vi "2D_voltage_mapping_lock-in-measurement_11_25_24.vi"() -> ()   [LabVIEW 2024]
uses:
  <vilib>/Utility/file.llb/Write Delimited Spreadsheet (string).vi
  <vilib>/Utility/file.llb/Write Delimited Spreadsheet (DBL).vi
  C:/Users/Public/OneDrive/Desktop/Keithley_2450_2470_1_4_0_LV2015_NewReadme2_2450-LV2015-1.4.0/Keithley 2450/Keithley 2450.lvlib
  archive/Keithley 24XX/Keithley 24XX.lvlib
  <vilib>/Analysis/NI_AALBase.lvlib
panel:
  out "current set voltage 2410":dbl
  out "Current set voltage 2450":dbl
  out "current voltage 2410":dbl=-5.417298089014366e-05 format="%0.4f"
  out "standard deviation current measured 2410":dbl=4.144039636185763e-09 format="%0.5e"
  out "mean current measured 2410":dbl=-4.484183666747521e-10 format="%0.5e"
  out "current voltage 2450":dbl=-2.554264496e-05 format="%0.4f"
  out "mean current measured 2450":dbl=-1.909496952e-09 format="%0.5e"
  out "standard deviation current measured 2450":dbl=9.060540822205692e-09 format="%0.5e"
  in  "VISA resource name 2410":refnum<visa-resource-name>="GPIB0::16::INSTR"
  in  "Serial Configuration":T1={"Baud Rate"=9600, "Parity"=0, "Data Bits"=8, "Stop Bits"=10, "Flow Control"=0} {"Flow Control" items=["None", "XON/XOFF", "RTS/CTS", "XON/XOFF & RTS/CTS", "DTR/DSR", "XON/XOFF & DTR/DSR"]; "Stop Bits" items=["1.0"=10, "1.5"=15, "2.0"=20]; "Data Bits" items=["7"=7, "8"=8]; "Parity" items=["None", "Odd", "Even", "Mark", "Space"]; "Baud Rate" items=["300"=300, "600"=600, "1200"=1200, "2400"=2400, "4800"=4800, "9600"=9600, "19200"=19200]}
  in  "Compliance  Level 2410":dbl=5e-08
  in  "Current Num Meas":i32=20 min=1 max=300000 step=1
  in  "VISA resource name 2450":refnum<visa-resource-name>="GPIB0::1::INSTR"
  in  "Current Compliance Limit (0.1) 2450":dbl=5e-08
  in  "ChB Parameter 1":u16(ring)=8 items=["X", "Y", "R", "Theta", "Frequency", "Noise", "Xh1", "Yh1", "Rh1", "Theta h1", "Xh2", "Yh2", "Rh2", "Theta h2"]
  in  "ChB Parameter 2":u16(ring)=9 items=["X", "Y", "R", "Theta", "Frequency", "Noise", "Xh1", "Yh1", "Rh1", "Theta h1", "Xh2", "Yh2", "Rh2", "Theta h2"]
  in  "ChA Parameter 2":u16(ring)=3 items=["X", "Y", "R", "Theta", "Frequency", "Noise", "Xh1", "Yh1", "Rh1", "Theta h1", "Xh2", "Yh2", "Rh2", "Theta h2"]
  in  "ChA Parameter 1":u16(ring)=2 items=["X", "Y", "R", "Theta", "Frequency", "Noise", "Xh1", "Yh1", "Rh1", "Theta h1", "Xh2", "Yh2", "Rh2", "Theta h2"]
  in  "Lock-In Num Avgs":i32=150
  out "错误输出":errorcluster
  in  "OE1022D 2":refnum<visa-resource-name>="COM4" caption="OE1022D"
  in  "ms to wait after move":u32=1000
  in  "Snake":bool
  in  "File to save to":path=path "D:/LabData/XiaoWang_Group_data_2024on/StackingTransitions/CrI3/round5_pfm_dualgate/11-14-4Lsample/RMCD/0T_after_m2T_map.txt"
  in  "Select Scan Type":u16(ring)=1 items=["line scan", "rectangular scan"]
  in  "scan points":i32
  in  "2410 end":i32
  in  "2450 end":i32
  in  "2410 start":i32
  in  "2450 start":i32
  in  "scan points":i32=30
  in  "2450 scan size":dbl=50.0 format="%.2f"
  in  "2410 scan size":dbl=50.0 format="%_2f"
  in  "2450 center":i32=25
  in  "2410 center":i32=25
  # "Scaning Setup"
  # "Rectangular Scan Parameters"
  # "Line Scan Parameters"
  # "Measurement Setup"
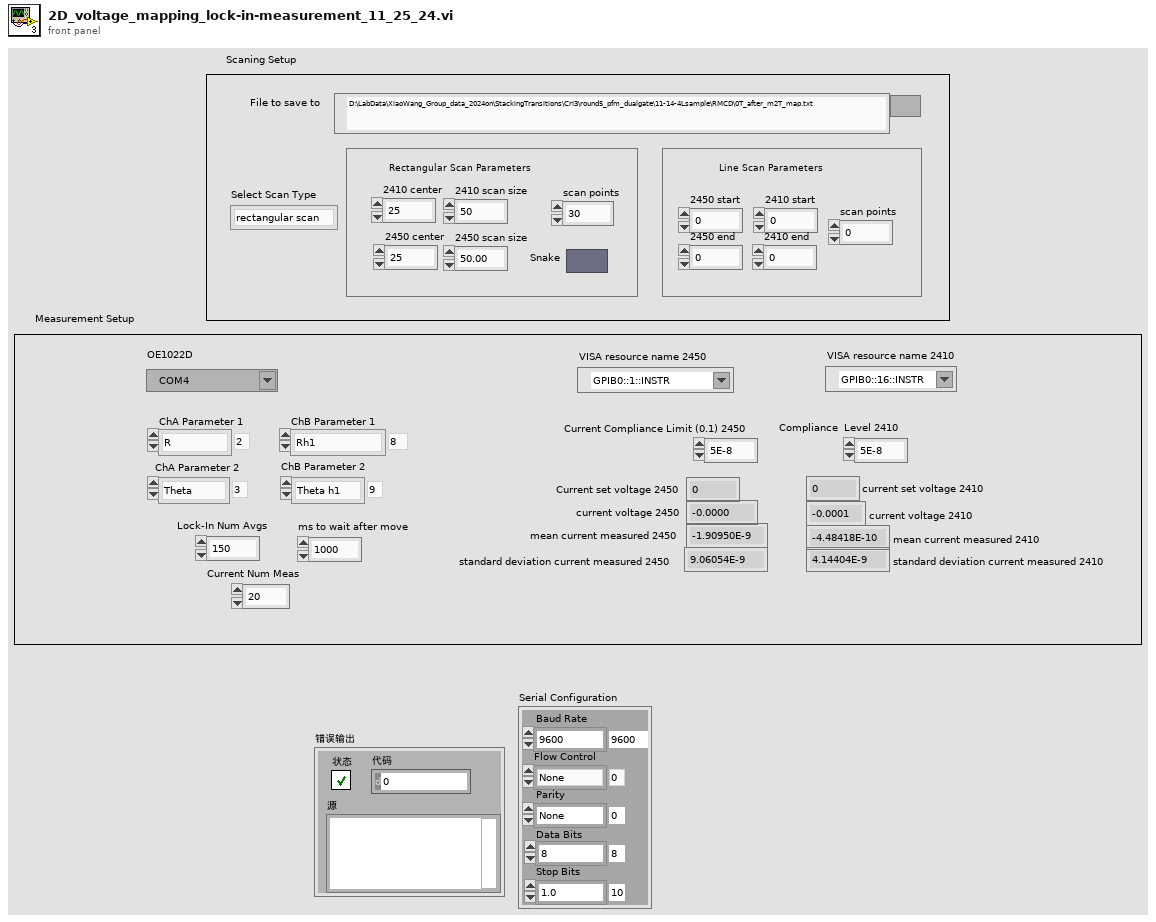
[diagram p1: front panel]
types:
  T1 = cluster{"Baud Rate":u32, "Parity":u16, "Data Bits":u16, "Stop Bits":u16, "Flow Control":u16}
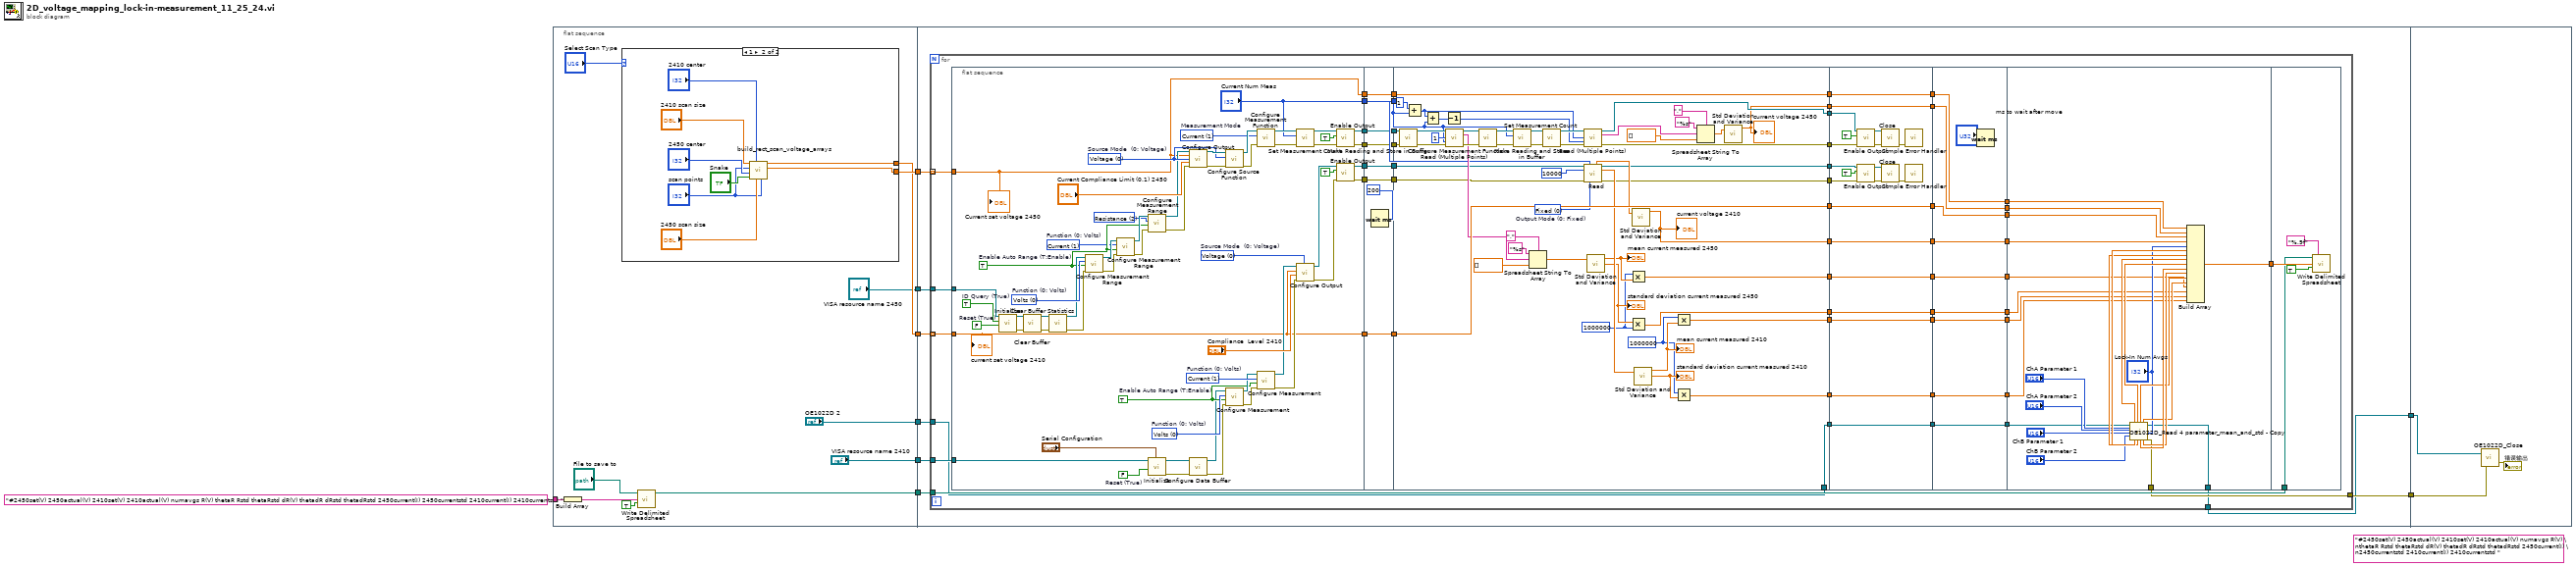
[diagram p0: block diagram]
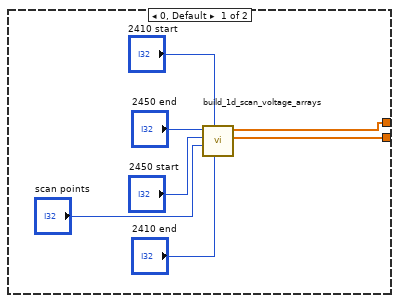
[diagram p2: hidden frame]
diagram:
  (unwired) "#2450set(V) 2450actual(V) 2410set(V) 2410actual(V) numavgs R(V) \nthetaR Rstd thetaRstd dR(V) thetadR dRstd thetadRstd 2450current(I) \n2450currentstd 2410current(I) 2410currentstd "
  n1 = flat-sequence {
    tunnel: [w16] -> w9
    tunnel: [w20] -> w8
    tunnel: [w12] -> w7
    tunnel: ["VISA resource name 2450"] -> w6
    tunnel: ["VISA resource name 2410"] -> w5
    tunnel: "#2450set(V) 2450actual(V) 2410set(V) 2410actual(V) numavgs R(V) thetaR Rstd thetaRstd dR(V) thetadR dRstd thetadRstd 2450current(I) 2450currentstd 2410current(I) 2410currentstd " -> [w11]
    tunnel: ["OE1022D 2"] -> w1
    tunnel: w9 -> [w43]
    tunnel: w8 -> [w42]
    tunnel: w7 -> [w41]
    tunnel: w6 -> [w40]
    tunnel: w5 -> [w39]
    tunnel: [w38] -> w3
    tunnel: [w37] -> w2
    tunnel: w1 -> [w36]
    tunnel: w3 -> [w277]
    tunnel: w2 -> [w276]
    frame #0 {
      n2 = Build Array(w11) -> (w17:string[])
      n3 = case shown="1" "Select Scan Type" {
        tunnel: [w21 w35] -> w20
        tunnel: [w22 w34] -> w16
        frame 0, Default {
          n4 = call "build_1d_scan_voltage_arrays.vi"("y end"="2410 end", "y start"="2410 start", "scan points"="scan points", "x start"="2450 start", "x end"="2450 end") -> ("y voltage array"=w21:dbl[], "x voltage array"=w22:dbl[])  [unwired: 5 in]
        }
        frame 1 {
          n5 = call "build_rect_scan_voltage_arrays.vi"("y scan points"="scan points", "y scan size"="2450 scan size", "x center"="2410 center", "Snake"="Snake", "y center"="2450 center", "x scan points"="scan points", "x scan size"="2410 scan size") -> ("y voltage array"=w35:dbl[], "x voltage array"=w34:dbl[])  [unwired: 3 in]
        }
      }
      n6 = call-poly <vilib>:"Write Delimited Spreadsheet.vi"("file path (dialog if empty)"="File to save to", "1D data"=w17, "append to file? (new file:F)"=TRUE) -> ("new file path (Not A Path if cancelled)"=w12:path)  [unwired: 11 in, 1 out]
    }
    frame #1 {
      n7 = for {
        tunnel: w43 -> [w97] mode=indexing
        tunnel: w42 -> [w96] mode=indexing
        tunnel: w41 -> [w92]
        tunnel: w40 -> [w91]
        tunnel: w39 -> [w90]
        tunnel: [w49] -> w38
        tunnel: [w48] -> w37
        tunnel: w36 -> [w44]
        n8 = flat-sequence {
          tunnel: w97 -> [w103]
          tunnel: w96 -> [w125]
          tunnel: [w103] -> w63
          tunnel: [w125] -> w61
          tunnel: w91 -> [w124]
          tunnel: w90 -> [w104]
          tunnel: [w102] -> w59
          tunnel: [w101] -> w57
          tunnel: ["Current Num Meas"] -> w55
          tunnel: [w99] -> w53
          tunnel: [w98] -> w51
          tunnel: w63 -> [w162]
          tunnel: [w162] -> w62
          tunnel: w61 -> [w161]
          tunnel: [w161] -> w60
          tunnel: w59 -> [w160]
          tunnel: [w160] -> w58
          tunnel: w57 -> [w159]
          tunnel: [w159] -> w56
          tunnel: w55 -> [w158]
          tunnel: [w158] -> w54
          tunnel: w53 -> [w157]
          tunnel: [w157] -> w52
          tunnel: w51 -> [w156]
          tunnel: [w156] -> w50
          tunnel: w62 -> [w215]
          tunnel: [w215] -> w89
          tunnel: w60 -> [w214]
          tunnel: [w214] -> w87
          tunnel: w58 -> [w211]
          tunnel: w56 -> [w210]
          tunnel: [w209] -> w85
          tunnel: [w208] -> w84
          tunnel: w54 -> [w172]
          tunnel: w52 -> [w174]
          tunnel: w50 -> [w173]
          tunnel: [w171] -> w83
          tunnel: [w170] -> w82
          tunnel: [w169] -> w79
          tunnel: [w168] -> w76
          tunnel: [w167] -> w73
          tunnel: [w166] -> w70
          tunnel: [w165] -> w67
          tunnel: [w164] -> w64
          tunnel: [w163] -> w45
          tunnel: w44 -> [w163]
          tunnel: w89 -> [w236]
          tunnel: [w236] -> w88
          tunnel: w87 -> [w235]
          tunnel: [w235] -> w86
          tunnel: w85 -> [w230]
          tunnel: w84 -> [w231]
          tunnel: w83 -> [w224]
          tunnel: w82 -> [w223]
          tunnel: [w222] -> w80
          tunnel: w79 -> [w222]
          tunnel: [w221] -> w77
          tunnel: w76 -> [w221]
          tunnel: [w220] -> w74
          tunnel: w73 -> [w220]
          tunnel: [w219] -> w71
          tunnel: w70 -> [w219]
          tunnel: [w218] -> w68
          tunnel: w67 -> [w218]
          tunnel: [w217] -> w65
          tunnel: w64 -> [w217]
          tunnel: [w216] -> w46
          tunnel: w45 -> [w216]
          tunnel: [w245] -> w94
          tunnel: w88 -> [w245]
          tunnel: w86 -> [w244]
          tunnel: [w244] -> w93
          tunnel: [w243] -> w81
          tunnel: w80 -> [w243]
          tunnel: [w242] -> w78
          tunnel: w77 -> [w242]
          tunnel: [w241] -> w75
          tunnel: w74 -> [w241]
          tunnel: [w240] -> w72
          tunnel: w71 -> [w240]
          tunnel: [w239] -> w69
          tunnel: w68 -> [w239]
          tunnel: [w238] -> w66
          tunnel: w65 -> [w238]
          tunnel: [w237] -> w47
          tunnel: w46 -> [w237]
          tunnel: [w271] -> w95
          tunnel: w94 -> [w258]
          tunnel: w93 -> [w259]
          tunnel: w81 -> [w262]
          tunnel: w78 -> [w261]
          tunnel: w75 -> [w257]
          tunnel: w72 -> [w256]
          tunnel: w69 -> [w255]
          tunnel: w66 -> [w254]
          tunnel: [w249] -> w49
          tunnel: [w248] -> w48
          tunnel: w47 -> [w247]
          tunnel: w95 -> [w274]
          tunnel: w92 -> [w272]
          frame #0 {
            w112 = FALSE  # Reset (True)
            w113 = u16 0 items=["Voltage", "Current"]  # Source Mode  (0: Voltage)
            w111 = TRUE  # Enable Auto Range (T:Enable)
            w119 = u16 1 items=["Volts", "Current", "Resistance"]  # Function (0: Volts)
            w118 = u16 0 items=["Volts", "Current", "Resistance"]  # Function (0: Volts)
            w127 = u16 2 items=["Volts", "Current", "Resistance"] ("Function (0: Volts)")
            w145 = u16 0 items=["Voltage", "Current"]  # Source Mode  (0: Voltage)
            w146 = u16 1 items=["Volts", "Current", "Auto Resistance", "Manual Resistance", "Digitize Voltage", "Digitize Current"]  # Measurement Mode
            w126 = TRUE  # Enable Auto Range (T:Enable)
            w123 = u16 1 items=["Volts", "Current", "Resistance"]  # Function (0: Volts)
            w147 = u16 0 items=["Volts", "Current", "Resistance"]  # Function (0: Volts)
            w143 = FALSE  # Reset (True)
            w148 = TRUE  # ID Query (True)
            n9 = call "Initialize.vi"("Reset (True)"=w143, "ID Query (True)"=w148, "VISA resource name"=w124) -> ("error out"=w141:errorcluster, "VISA resource name out"=w142:refnum<visa-resource-name>)  [unwired: 7 in]
            n10 = call "Clear Buffer.vi"("VISA resource name"=w142, "error in (no error)"=w141) -> ("VISA resource name out"=w140:refnum<visa-resource-name>, "error out"=w137:errorcluster)  [unwired: 12 in]
            n11 = call "Clear Buffer Statistics.vi"("VISA resource name"=w140, "error in (no error)"=w137) -> ("VISA resource name out"=w139:refnum<visa-resource-name>, "error out"=w138:errorcluster)  [unwired: 12 in]
            n12 = call "Configure Measurement Range.vi"("error in (no error)"=w138, "Enable Auto Range (T:Enable)"=w126, "Function (0: Volts)"=w147, "VISA resource name"=w139) -> ("error out"=w150:errorcluster, "VISA resource name out"=w149:refnum<visa-resource-name>)  [unwired: 6 in]
            n13 = call "Configure Measurement Range.vi"("error in (no error)"=w150, "Enable Auto Range (T:Enable)"=w126, "Function (0: Volts)"=w123, "VISA resource name"=w149) -> ("error out"=w130:errorcluster, "VISA resource name out"=w131:refnum<visa-resource-name>)  [unwired: 6 in]
            n14 = call "Configure Measurement Range.vi"("error in (no error)"=w130, "Enable Auto Range (T:Enable)"=w126, "Function (0: Volts)"=w127, "VISA resource name"=w131) -> ("error out"=w129:errorcluster, "VISA resource name out"=w128:refnum<visa-resource-name>)  [unwired: 6 in]
            n15 = call "Initialize.vi"("Serial Configuration"="Serial Configuration", "Reset (True)"=w112, "VISA resource name"=w104) -> ("error out"=w107:errorcluster, "VISA resource name out"=w108:refnum<visa-resource-name>)  [unwired: 7 in]
            n16 = call "Configure Output.vi"("VISA resource name"=w128, "Source Level (0)"=w125, "Source Mode  (0: Voltage)"=w145, "Source Limit Level (0.1)"="Current Compliance Limit (0.1) 2450", "error in (no error)"=w129) -> ("VISA resource name out"=w151:refnum<visa-resource-name>, "error out"=w152:errorcluster)  [unwired: 9 in]
            n17 = call "Configure Data Buffer.vi"("error in (no error)"=w107, "VISA resource name"=w108) -> ("error out"=w106:errorcluster, "VISA resource name out"=w105:refnum<visa-resource-name>)  [unwired: 8 in]
            n18 = call "Configure Source Function.vi"("error in (no error)"=w152, "Function (0: Volts)"=w145, "VISA resource name"=w151) -> ("error out"=w153:errorcluster, "VISA resource name out"=w154:refnum<visa-resource-name>)  [unwired: 7 in]
            n19 = call "Configure Measurement.vi"("error in (no error)"=w106, "Enable Auto Range (T:Enable)"=w111, "Function (0: Volts)"=w118, "VISA resource name"=w105) -> ("error out"=w114:errorcluster, "VISA resource name out"=w115:refnum<visa-resource-name>)  [unwired: 6 in]
            n20 = call "Configure Measurement.vi"("error in (no error)"=w114, "Enable Auto Range (T:Enable)"=w111, "Function (0: Volts)"=w119, "VISA resource name"=w115) -> ("error out"=w109:errorcluster, "VISA resource name out"=w110:refnum<visa-resource-name>)  [unwired: 6 in]
            n21 = call "Configure Measurement Function.vi"("error in (no error)"=w153, "Function (0: Volts)"=w146, "VISA resource name"=w154) -> ("error out"=w134:errorcluster, "VISA resource name out"=w133:refnum<visa-resource-name>)  [unwired: 7 in]
            n22 = call "Set Measurement Count.vi"("error in (no error)"=w134, "Measurement Count"="Current Num Meas", "VISA resource name"=w133) -> ("error out"=w135:errorcluster, "VISA resource name out"=w136:refnum<visa-resource-name>)  [unwired: 7 in]
            n23 = call "Configure Output.vi"("Source Mode  (0: Voltage)"=w113, "error in (no error)"=w109, "Compliance  Level (0.1)"="Compliance  Level 2410", "Output Level (0)"=w103, "VISA resource name"=w110) -> ("error out"=w122:errorcluster, "VISA resource name out"=w121:refnum<visa-resource-name>)  [unwired: 5 in]
            n24 = call "Enable Output.vi"("error in (no error)"=w135, "Enable Output (T: Enable)"=TRUE, "VISA resource name"=w136) -> ("error out"=w101:errorcluster, "VISA resource name out"=w102:refnum<visa-resource-name>)  [unwired: 7 in]
            n25 = call "Enable Output.vi"("error in (no error)"=w122, "Enable Output (T: Enable)"=TRUE, "VISA resource name"=w121) -> ("error out"=w98:errorcluster, "VISA resource name out"=w99:refnum<visa-resource-name>)  [unwired: 7 in]
            "Current set voltage 2450" <- w125
            "current set voltage 2410" <- w103
          }
          frame #1 {
            n26 = Wait (ms)(milliseconds to wait=u32 200 ("Start Index (1)")) -> ()  [unwired: 1 out]
          }
          frame #2 {
            w190 = 1000000 ("Timeout (10000 ms)")
            w201 = 1000000 ("Timeout (10000 ms)")
            w206 = u16 0 items=["Fixed", "Sweep", "List"]  # Output Mode (0: Fixed)
            n27 = call "Make Reading and Store in Buffer.vi"("VISA resource name"=w211, "error in (no error)"=w210) -> ("VISA resource name out"=w199:refnum<visa-resource-name>, "error out"=w200:errorcluster)  [unwired: 12 in]
            n28 = Add(x=u32 1 ("Start Index (1)"), y=w172) -> (x+y=w176:u32)
            n29 = Add(x=w176, y=w172) -> (x+y=w177:u32)
            n30 = Decrement(x=w177) -> (x-1=w175:u32)
            n31 = call "Read (Multiple Points).vi"("VISA resource name"=w199, "Start Index (1)"=u32 1, "End Index (1)"=w172, "error in (no error)"=w200) -> ("VISA resource name out"=w213:refnum<visa-resource-name>, "Data out"=w194:string, "error out"=w212:errorcluster)  [unwired: 9 in]
            n32 = call "Configure Measurement Function.vi"("error in (no error)"=w212, "VISA resource name"=w213) -> ("error out"=w185:errorcluster, "VISA resource name out"=w189:refnum<visa-resource-name>)  [unwired: 8 in]
            n33 = call "Set Measurement Count.vi"("error in (no error)"=w185, "Measurement Count"=w172, "VISA resource name"=w189) -> ("error out"=w186:errorcluster, "VISA resource name out"=w184:refnum<visa-resource-name>)  [unwired: 7 in]
            n34 = Spreadsheet String To Array(delimiter (Tab)=",", format string="%s", spreadsheet string=w194, array type (2D Dbl)=dbl[] []) -> (array=w193:dbl[])
            n35 = call "Make Reading and Store in Buffer.vi"("VISA resource name"=w184, "error in (no error)"=w186) -> ("VISA resource name out"=w188:refnum<visa-resource-name>, "error out"=w187:errorcluster)  [unwired: 12 in]
            n36 = call "Read (Multiple Points).vi"("VISA resource name"=w188, "Start Index (1)"=w176, "End Index (1)"=w175, "error in (no error)"=w187) -> ("VISA resource name out"=w209:refnum<visa-resource-name>, "Data out"=w180:string, "error out"=w208:errorcluster)  [unwired: 9 in]
            n37 = call-poly "Read.vi"("VISA resource name"=w174, "Sample Count (1)"=w172, "Timeout (10000 ms)"=10000, "error in (no error)"=w173, "Output Mode (0: Fixed)"=w206) -> ("Voltage"=w204:sgl[], "VISA resource name out"=w171:refnum<visa-resource-name>, "Current"=w205:sgl[], "error out"=w170:errorcluster)  [unwired: 4 in, 3 out]
            n38 = call <vilib>:"Std Deviation and Variance.vi"("X"=w193) -> ("mean"=w191:dbl, "standard deviation"=w192:dbl)  [unwired: 1 in, 1 out]
            "mean current measured 2450" <- w191
            "standard deviation current measured 2450" <- w192
            n39 = Multiply(x=w190, y=w191) -> (x*y=w167:dbl)
            n40 = Multiply(x=w192, y=w190) -> (x*y=w166:dbl)
            n41 = call <vilib>:"Std Deviation and Variance.vi"("X"=w204) -> ("mean"=w168:dbl)  [unwired: 1 in, 2 out]
            "current voltage 2410" <- w168
            n42 = call <vilib>:"Std Deviation and Variance.vi"("X"=w205) -> ("mean"=w202:dbl, "standard deviation"=w203:dbl)  [unwired: 1 in, 1 out]
            "mean current measured 2410" <- w202
            "standard deviation current measured 2410" <- w203
            n43 = Multiply(x=w201, y=w202) -> (x*y=w165:dbl)
            n44 = Multiply(x=w201, y=w203) -> (x*y=w164:dbl)
            n45 = Spreadsheet String To Array(delimiter (Tab)=",", format string="%s", spreadsheet string=w180, array type (2D Dbl)=dbl[] []) -> (array=w179:dbl[])
            n46 = call <vilib>:"Std Deviation and Variance.vi"("X"=w179) -> ("mean"=w169:dbl)  [unwired: 1 in, 2 out]
            "current voltage 2450" <- w169
          }
          frame #3 {
            n47 = call "Enable Output.vi"("error in (no error)"=w231, "Enable Output (T: Enable)"=TRUE, "VISA resource name"=w230) -> ("error out"=w233:errorcluster, "VISA resource name out"=w234:refnum<visa-resource-name>)  [unwired: 7 in]
            n48 = call "Enable Output.vi"("error in (no error)"=w223, "Enable Output (T: Enable)"=TRUE, "VISA resource name"=w224) -> ("error out"=w227:errorcluster, "VISA resource name out"=w228:refnum<visa-resource-name>)  [unwired: 7 in]
            n49 = call "Close.vi"("error in (no error)"=w233, "VISA resource name"=w234) -> ("error out"=w232:errorcluster)  [unwired: 9 in]
            n50 = call "Close.vi"("error in (no error)"=w227, "VISA resource name"=w228) -> ("error out"=w226:errorcluster)  [unwired: 9 in]
            n51 = call <vilib>:"Simple Error Handler.vi"("error in (no error)"=w232) -> ()  [unwired: 4 in, 5 out]
            n52 = call <vilib>:"Simple Error Handler.vi"("error in (no error)"=w226) -> ()  [unwired: 4 in, 5 out]
          }
          frame #4 {
            n53 = Wait (ms)(milliseconds to wait="ms to wait after move") -> ()  [unwired: 1 out]
          }
          frame #5 {
            n54 = call "OE1022D_Read 4 parameter_mean_and_std - Copy.vi"("VISA resource name"=w247, "ChA Parameter 1"="ChA Parameter 1", "ChA Parameter 2"="ChA Parameter 2", "ChB Parameter 1"="ChB Parameter 1", "ChB Parameter 2"="ChB Parameter 2", "Num Averages"="Lock-In Num Avgs") -> ("Measurement STD"=w268:dbl, "Measurement"=w270:dbl, "Measurement STD 2"=w267:dbl, "Measurement 2"=w269:dbl, "Measurement STD 3"=w264:dbl, "Measurement 3"=w266:dbl, "Measurement STD 4"=w263:dbl, "Measurement 4"=w265:dbl, "VISA resource name out"=w248:refnum<visa-resource-name>, "error out"=w249:errorcluster)  [unwired: 4 in]
            n55 = Build Array(w259, w262, w258, w261, "Lock-In Num Avgs", w270, w269, w268, w267, w266, w265, w264, w263, w257, w256, w255, w254) -> (w271:dbl[])
          }
          frame #6 {
            n56 = call-poly <vilib>:"Write Delimited Spreadsheet.vi"("file path (dialog if empty)"=w272, "format (%.3f)"="%.9f", "1D data"=w274, "append to file? (new file:F)"=TRUE) -> ()  [unwired: 10 in, 2 out]
          }
        }
      }
    }
    frame #2 {
      n57 = call "OE1022D_Close.vi"("错误输入（无错误）"=w277, "VISA resource name"=w276) -> ("错误输出"=→"错误输出":errorcluster)  [unwired: 1 in]
    }
  }
